vi "Generate.vi"(0 "reference in":refnum<class "Python.lvclass">, 1 "Path":path, 3 "Classes":T1[](array[typedef]), 5 "error in (no error)":errorcluster) -> (14 "reference out":refnum<class "Python.lvclass">, 19 "error out":errorcluster)   [LabVIEW 2018, in "Python.lvclass"]
uses:
  Python.lvclass
  Executer_class/typedefs/ClassDescription.ctl
  Executer_class/typedefs/MethodDescription.ctl
  Executer_class/Executer.lvclass
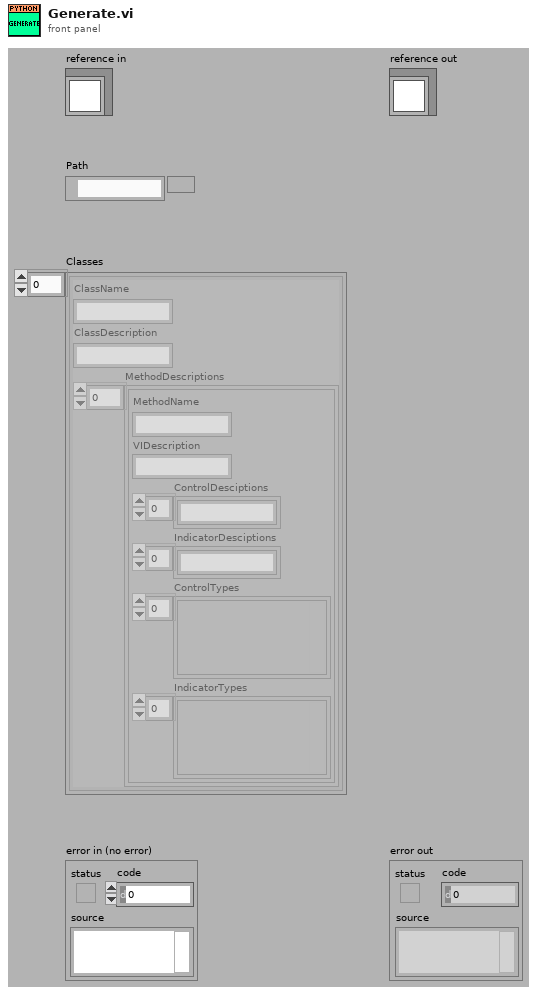
[diagram p1: front panel]
types:
  T1 = typedef "Executer.lvclass/ClassDescription.ctl" = cluster{"ClassName":string, "ClassDescription":string, "MethodDescriptions":T2[]}
  T2 = typedef "Executer.lvclass/MethodDescription.ctl" = cluster{"MethodName":string, "VIDescription":string, "ControlDesciptions":string[], "IndicatorDesciptions":string[], "ControlTypes":variant[], "IndicatorTypes":variant[]}
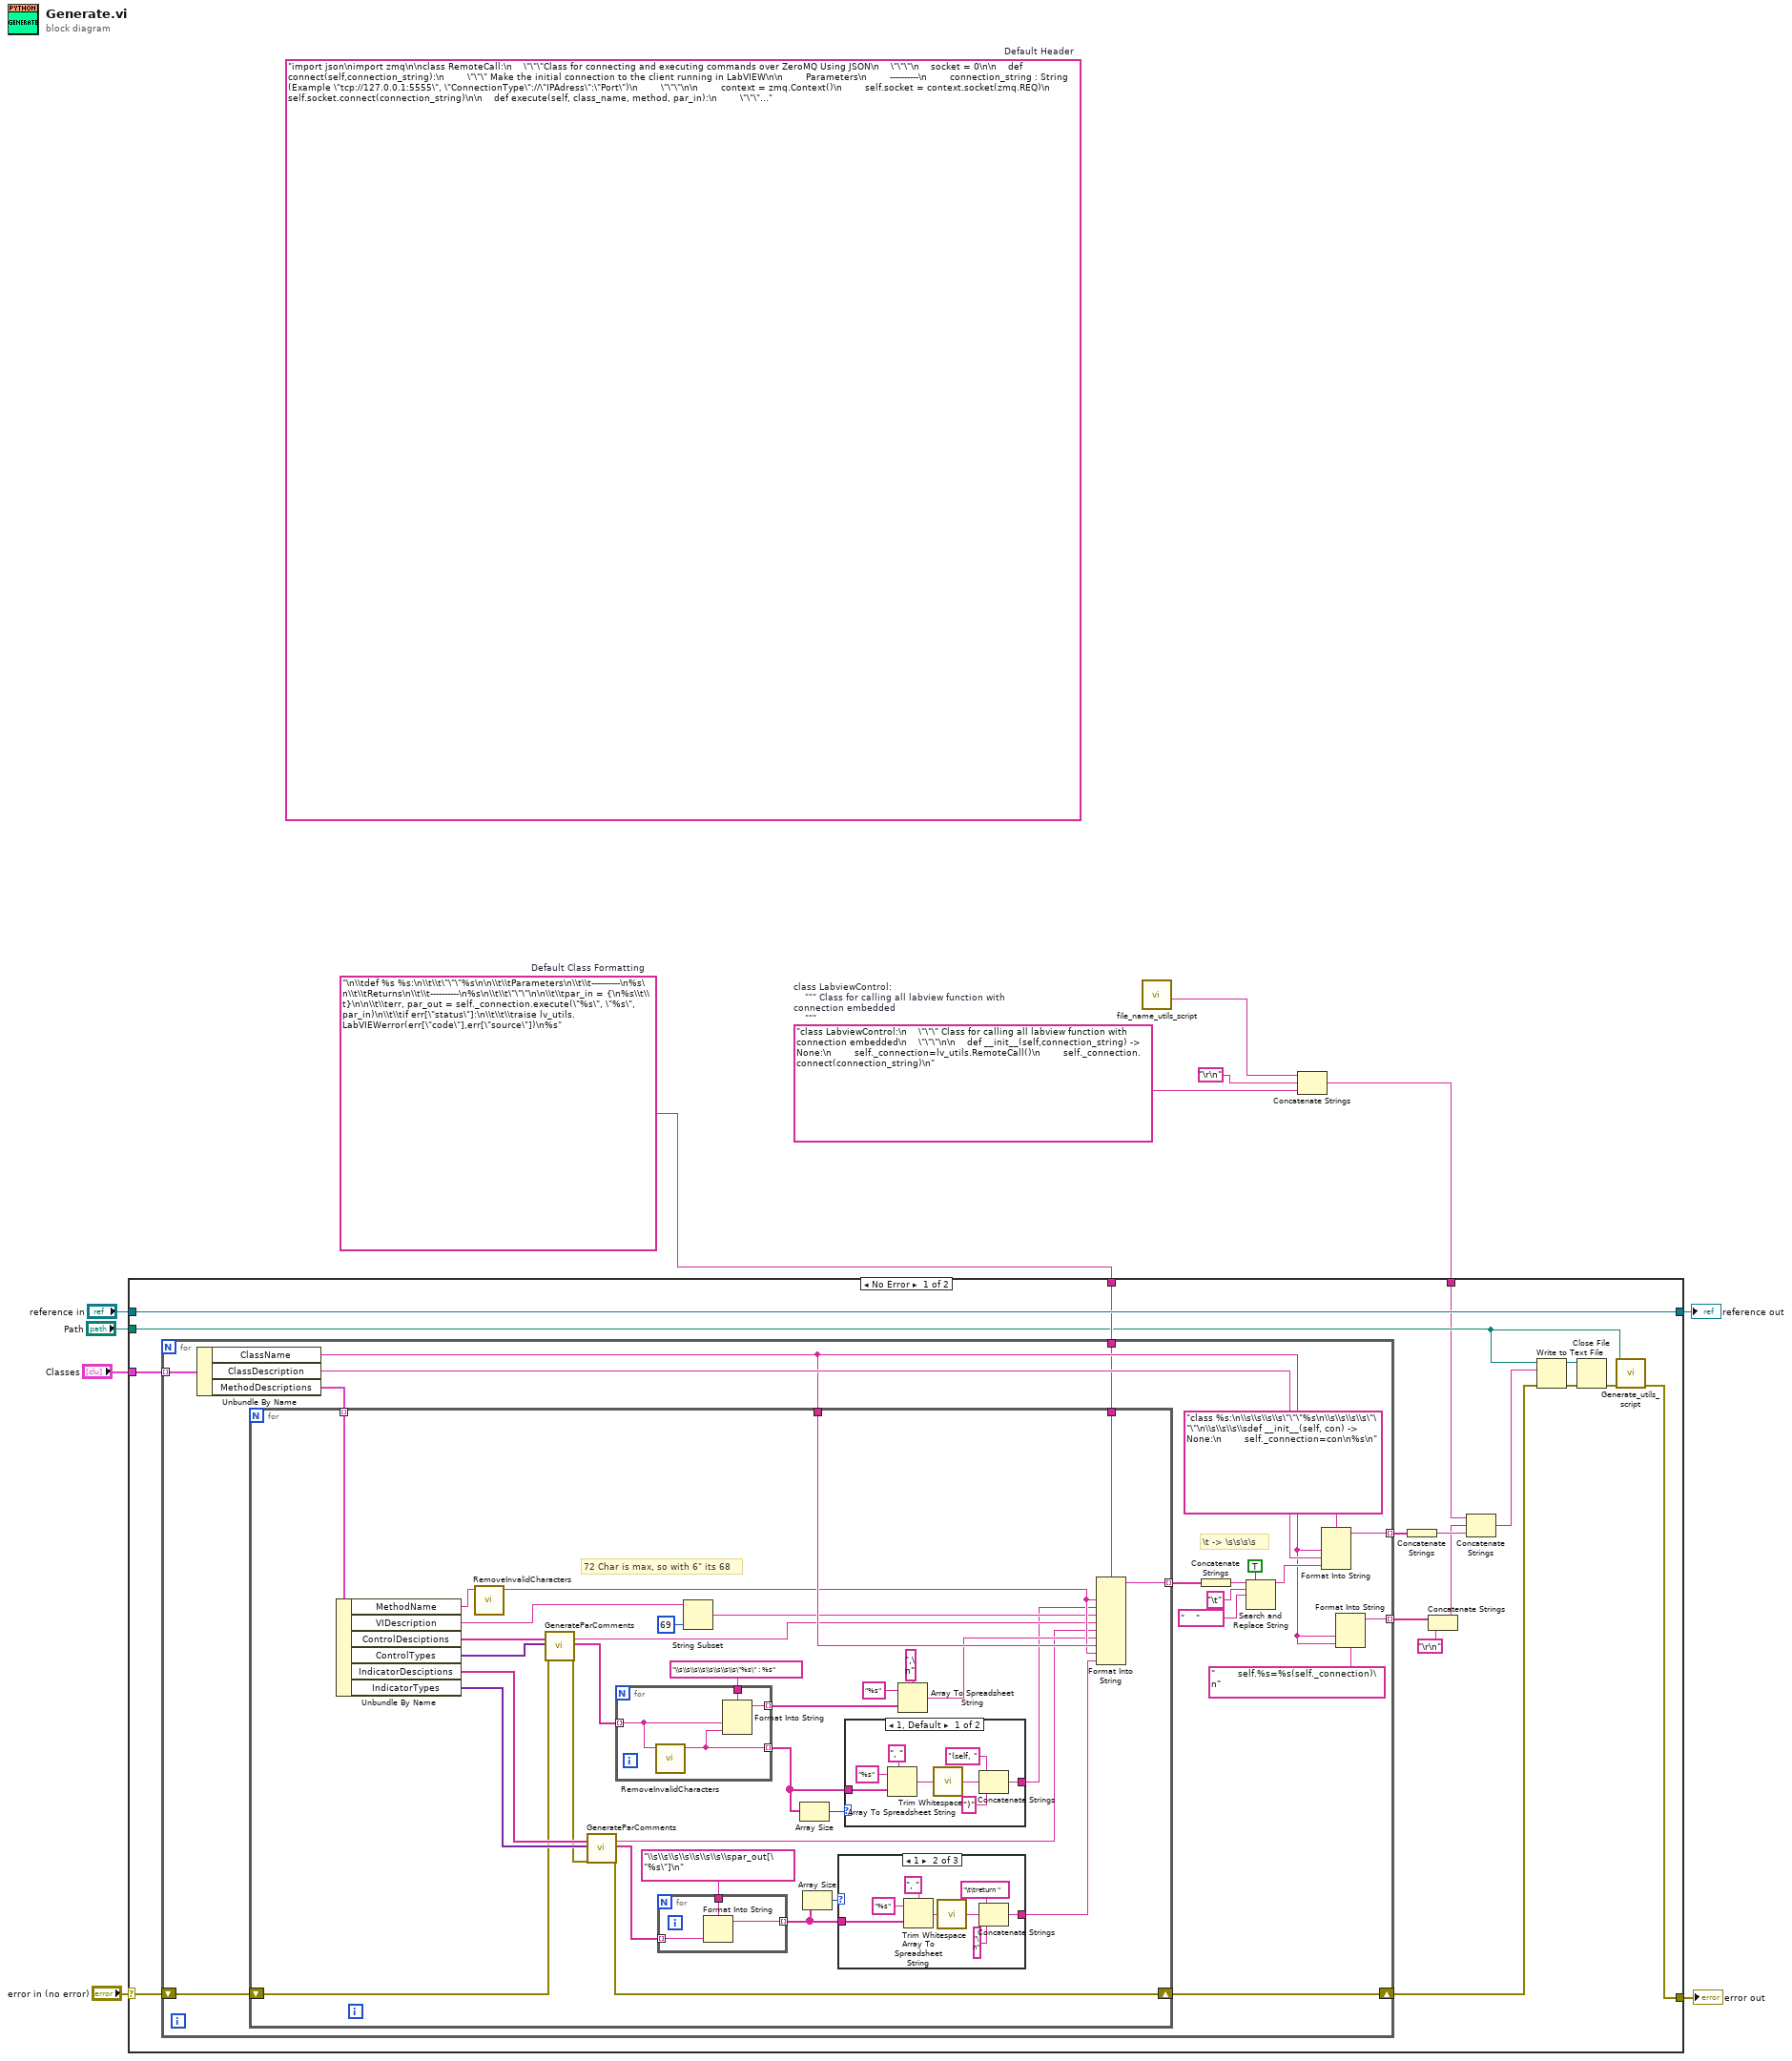
[diagram p0: block diagram]
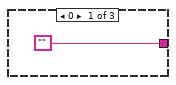
[diagram p2: hidden frame]
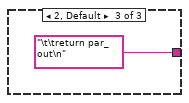
[diagram p3: hidden frame]
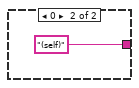
[diagram p4: hidden frame]
diagram:
  w4 = "class LabviewControl:\n    \"\"\" Class for calling all labview function with connection embedded\n    \"\"\"\n\n    def __init__(self,connection_string) -> None:\n        self._connection=lv_utils.RemoteCall()\n        self._connection.connect(connection_string)\n"  # class LabviewControl:     """ Class for calling all labview function with connection embedded     """      def __init__(self,connection_string) -> None:         self._connection=lv_utils.RemoteCall()         self._connection.connect(connection_string)
  w5 = "\n\\tdef %s %s:\n\\t\\t\"\"\"%s\n\n\\t\\tParameters\n\\t\\t----------\n%s\n\\t\\tReturns\n\\t\\t----------\n%s\n\\t\\t\"\"\"\n\n\\t\\tpar_in = {\n%s\\t\\t}\n\n\\t\\terr, par_out = self._connection.execute(\"%s\", \"%s\", par_in)\n\\t\\tif err[\"status\"]:\n\\t\\t\\traise lv_utils.LabVIEWerror(err[\"code\"],err[\"source\"])\n%s"  # Default Class Formatting
  (unwired) "import json\nimport zmq\n\nclass RemoteCall:\n    \"\"\"Class for connecting and executing commands over ZeroMQ Using JSON\n    \"\"\"\n    socket = 0\n\n    def connect(self,connection_string):\n        \"\"\" Make the initial connection to the client running in LabVIEW\n\n        Parameters\n        ----------\n        connection_string : String (Example \"tcp://127.0.0.1:5555\", \"ConnectionType\"://\"IPAdress\":\"Port\")\n        \"\"\"\n\n        context = zmq.Context()\n        self.socket = context.socket(zmq.REQ)\n        self.socket.connect(connection_string)\n\n    def execute(self, class_name, method, par_in):\n        \"\"\" Execute the Method by serializing inputs sending it over, and deserializing the result\n        \"\"\"\n        data_2_send = \"{ \\\"Command\\\":\\\"Execute\\\" }\\x17{\\\"ClassLabel\\\":\\\"%s\\\",\\\"Method\\\":\\\"%s\\\"}\\x17%s\" % (class_name, method, json.dumps({\"In\": par_in}))\n        self.socket.send_string (data_2_send)\n        message = self.socket.recv()\n        parts = message.split(chr(0x17).encode())\n        return json.loads(parts[1]), json.loads(parts[0])\n\nclass LabVIEWerror(Exception):\n    \"\"\"Base class for all LabVIEW errors\n\n    Attributes\n    ----------\n    code: error code for testing which error happend\n    source: source of the error\n    \"\"\"\n    def __init__(self, *args: object) -> None:\n        self.code = self.args[0]\n        self.source = self.args[1]\n        super().__init__(*args)\n\n    def __str__(self) -> str:\n        return f\"LabVIEW Error with code: {self.code} source: {self.source}\"\n\nclass LabviewControl:\n    \"\"\" Class for calling all labview function with connection embedded\n    \"\"\"\n\n    def __init__(self,connection_string) -> None:\n        self._connection=RemoteCall()\n        self._connection.connect(connection_string)\n"  # Default Header
  n1 = call "file_name_utils_script.vi"() -> ("import statement"=w2:string)  [unwired: 10 in, 1 out]
  n2 = Concatenate Strings(w2, "\r\n", w4) -> (w3:string)
  n3 = case shown="No Error" "error in (no error)" {
    selector: "error in (no error)" -> [w21 w105]
    tunnel: [w13 w105] -> w10
    tunnel: [w22 w104] -> w8
    tunnel: "reference in" -> [w22 w104]
    tunnel: "Classes" -> [w20 _]
    tunnel: "Path" -> [w14 _]
    tunnel: w3 -> [w12 _]
    tunnel: w5 -> [w16 _]
    frame No Error {
      n4 = for {
        tunnel: [w45] -> w28 mode=indexing
        tunnel: w20 -> [w35] mode=indexing
        shift-right: [w37] -> w23
        shift-left: w21 -> [w36]
        tunnel: [w30] -> w19 mode=indexing
        tunnel: w16 -> [w29]
        # "\\t -> \\s\\s\\s\\s"
        n5 = Unbundle By Name(w35) -> ("ClassName"=w31:string, "ClassDescription"=w34:string, "MethodDescriptions"=w33:T2[])
        n6 = for {
          tunnel: [w77] -> w44 mode=indexing
          tunnel: w31 -> [w76]
          shift-right: [w51] -> w37
          shift-left: w36 -> [w53]
          tunnel: w33 -> [w50] mode=indexing
          tunnel: w29 -> [w48]
          # "72 Char is max, so with 6\" its 68"
          n7 = Unbundle By Name(w50) -> ("MethodName"=w49:string, "VIDescription"=w65:string, "ControlDesciptions"=w64:string[], "ControlTypes"=w63:variant[], "IndicatorDesciptions"=w54:string[], "IndicatorTypes"=w55:variant[])
          n8 = call "RemoveInvalidCharacters.vi"("string in"=w49) -> ("string out"=w75:string)  [unwired: 10 in]
          n9 = call "GenerateParComments.vi"("Desciptions"=w64, "Types"=w63, "error in (no error)"=w53) -> ("DescriptionString"=w62:string, "Names"=w60:string[], "error out"=w52:errorcluster)  [unwired: 14 in]
          n10 = call "GenerateParComments.vi"("Desciptions"=w54, "Types"=w55, "error in (no error)"=w52) -> ("DescriptionString"=w61:string, "Names"=w59:string[], "error out"=w51:errorcluster)  [unwired: 14 in]
          n11 = for {
            tunnel: [w94] -> w69 mode=indexing
            tunnel: [w93] -> w57 mode=indexing
            tunnel: w60 -> [w92] mode=indexing
            tunnel: "\\s\\s\\s\\s\\s\\s\\s\\s\"%s\" : %s" ("string") -> [w91]
            n12 = call "RemoveInvalidCharacters.vi"("string in"=w92) -> ("string out"=w93:string)  [unwired: 10 in]
            n13 = Format Into String(format string=w91, w92, w93) -> (resulting string=w94:string)  [unwired: 2 in, 1 out]
          }
          n14 = for {
            tunnel: [w90] -> w70 mode=indexing
            tunnel: w59 -> [w89] mode=indexing
            tunnel: "\\s\\s\\s\\s\\s\\s\\s\\spar_out[\"%s\"]\n" ("string") -> [w88]
            n15 = Format Into String(format string=w88, w89) -> (resulting string=w90:string)  [unwired: 2 in, 1 out]
          }
          n16 = String Subset(string=w65, length (rest)=69 ("length (rest)")) -> (substring=w74:string)  [unwired: 1 in]
          n17 = Array Size(array=w57) -> (size(s)=w56:i32)
          n18 = Array Size(array=w70) -> (size(s)=w72:i32)
          n19 = case shown="1" w72 {
            tunnel: ["" w86 "\t\treturn par_out\n" ("string")] -> w71
            tunnel: w70 -> [_ w80 _]
            frame 0 {
            }
            frame 1 {
              n20 = Array To Spreadsheet String(delimiter (Tab)=", ", array=w80, 3:"%s" ("format string")) -> (spreadsheet string=w81:string)
              n21 = call <vilib>:"Trim Whitespace.vi"("string"=w81) -> ("trimmed string"=w79:string)  [unwired: 1 in]
              n22 = Concatenate Strings("\t\treturn " ("string"), w79, "\n" ("delimiter (Tab)")) -> (w86:string)
            }
            frame 2, Default {
            }
          }
          n23 = case shown="1, Default" w56 {
            tunnel: [w95 "(self)" ("string")] -> w58
            tunnel: w57 -> [w96 _]
            frame 1, Default {
              n24 = Array To Spreadsheet String(delimiter (Tab)=", ", array=w96, 3:"%s" ("format string")) -> (spreadsheet string=w99:string)
              n25 = call <vilib>:"Trim Whitespace.vi"("string"=w99) -> ("trimmed string"=w101:string)  [unwired: 1 in]
              n26 = Concatenate Strings("(self, " ("string"), w101, ")" ("string")) -> (w95:string)
            }
            frame 0 {
            }
          }
          n27 = Array To Spreadsheet String(delimiter (Tab)=",\n", array=w69, 3:"%s" ("format string")) -> (spreadsheet string=w66:string)
          n28 = Format Into String(format string=w48, w75, w58, w74, w62, w61, w66, w76, w75, w71) -> (resulting string=w77:string)  [unwired: 2 in, 1 out]
        }
        n29 = Concatenate Strings(w44) -> (w43:string)
        n30 = Search and Replace String(replace all?=TRUE ("replace all? (F)"), input string=w43, search string="\t", replace string="    " ("search string")) -> (result string=w38:string)  [unwired: 4 in, 3 out]
        n31 = Format Into String(format string="class %s:\n\\s\\s\\s\\s\"\"\"%s\n\\s\\s\\s\\s\"\"\"\n\\s\\s\\s\\sdef __init__(self, con) -> None:\n        self._connection=con\n%s\n", w31, w34, w38) -> (resulting string=w45:string)  [unwired: 2 in, 1 out]
        n32 = Format Into String(format string="        self.%s=%s(self._connection)\n", w31, w31) -> (resulting string=w30:string)  [unwired: 2 in, 1 out]
      }
      n33 = Concatenate Strings(w28) -> (w27:string)
      n34 = Concatenate Strings(w19, "\r\n") -> (w18:string)
      n35 = Concatenate Strings(w12, w18, w27) -> (w26:string)
      n36 = Write to Text File(file (use dialog)=w14, text=w26, error in=w23) -> (refnum out=w25:refnum<file>, error out=w24:errorcluster)  [unwired: 1 in, 1 out]
      n37 = Close File(refnum=w25, error in=w24) -> (error out=w15:errorcluster)  [unwired: 1 out]
      n38 = call "Generate_utils_script.vi"("error in (no error)"=w15, "Path"=w14) -> ("error out"=w13:errorcluster)  [unwired: 9 in]
    }
    frame Error {
    }
  }
  "error out" <- w10
  "reference out" <- w8
